vi "Save Start-up Configuration.vi"() -> ()   [LabVIEW 2015]
uses:
  Start-up Configuration.ctl
  Module Types.ctl
  <vilib>/Utility/config.llb/NI_LVConfig.lvlib
panel:
  in  "File path":path=path "C:/Data/Config/start-up.cfg"
  in  "Initial Configuration":T1={"Load Modules"=[enum."Pulse Controller", enum."Monitor Controller", enum."NI-DAQmx", enum."NI-Scope", enum."Red Pitaya Digitizer", enum."VISA Device", enum."Red Piataya Lockin", enum."Integrate Pulse", enum."Lockin Processor"]}
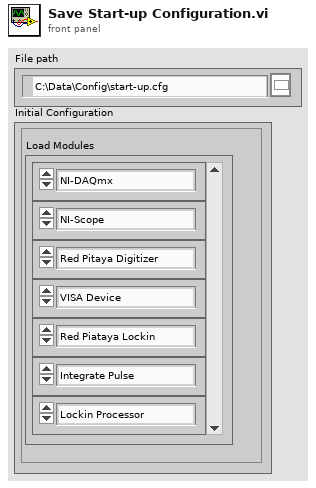
[diagram p1: front panel]
types:
  T1 = typedef "Start-up Configuration.ctl" = cluster{"Load Modules":T2[]}
  T2 = typedef "Module Types.ctl" = enum16{"NONE", "NI-DAQmx", "NI-Scope", "Red Pitaya Digitizer", "GaGe", "VISA Device", "Red Piataya Lockin", "Monitor Controller", "Pulse Controller", "Integrate Pulse", "Lockin Processor"}
  T3 = typedef "NI_LVConfig.lvlib/Config Data RefNum.ctl" = refnum<k1>
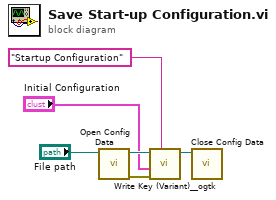
[diagram p0: block diagram]
diagram:
  n1 = call <vilib>:"Open Config Data.vi"("configuration file path"="File path") -> ("error out"=w5:errorcluster, "refnum"=w4:T3)  [unwired: 8 in, 1 out]
  n2 = call <userlib>:"Write Key (Variant)__ogtk.vi"("section"="Startup Configuration", "error in (no error)"=w5, "key-value"="Initial Configuration", "refnum"=w4) -> ("refnum out"=w6:T3)  [unwired: 6 in, 1 out]
  n3 = call <vilib>:"Close Config Data.vi"("refnum"=w6) -> ()  [unwired: 9 in, 2 out]
